vi "DeQ.vi"(10 "Msg Q":refnum<data-value>) -> (0 "error out":errorcluster, 2 "Msg":refnum<class "Msg.lvclass">)   [LabVIEW 2021, in "LVCAM.lvlib" / "Msg Q.lvclass"]
uses:
  Msg Q.lvclass
  Msg/Msg.lvclass
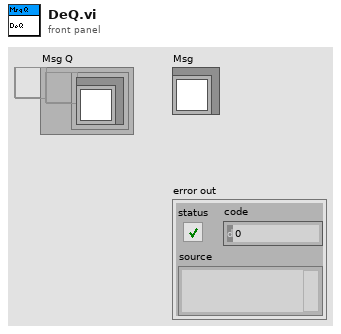
[diagram p1: front panel]
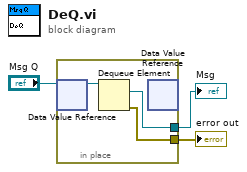
[diagram p0: block diagram]
diagram:
  n1 = in-place {
    in-place-border: [w5] -> w1
    in-place-border: [w4] -> w2
    n2 = in-place-dvr #1("Msg Q") -> (w6:refnum<queue>)  [unwired: 1 out]
    n3 = Dequeue Element(queue=w6) -> (element=w4:refnum<class "Msg.lvclass">, error out=w5:errorcluster)  [unwired: 2 in, 2 out]
    n4 = in-place-dvr #1() -> ()  [unwired: 1 in, 2 out]
  }
  "Msg" <- w2
  "error out" <- w1
